vi "GetInfo.vi"(8 "error in (no error)":errorcluster caption="错误输入（无错误）", 11 "XYPlot 输入":refnum<class "TrendPlot.lvclass">) -> (0 "error out":errorcluster caption="错误输出", 2 "通道变更":bool, 3 "XYPlot 输出":refnum<class "TrendPlot.lvclass">)   [LabVIEW 2018, in "DataDisplay.lvlib" / "TrendPlot.lvclass"]
uses:
  TrendPlot.lvclass
  TrendPlot.lvclass/TrendPlot.ctl
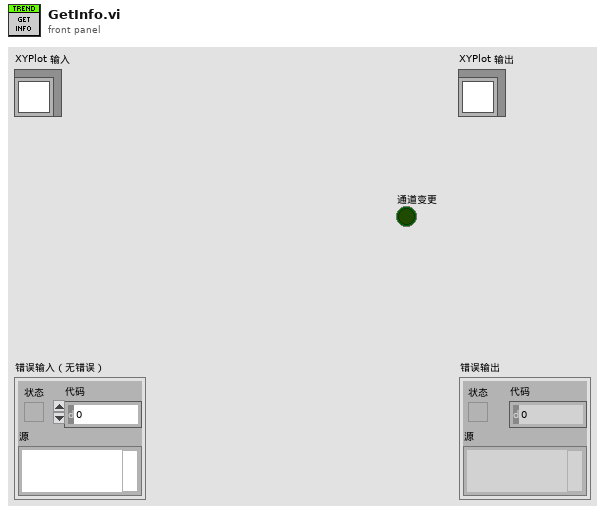
[diagram p1: front panel]
types:
  T1 = typedef "DataDisplay.lvlib/DD_CommandQ.ctl" = refnum<queue>
  T2 = typedef "DataDisplay.lvlib/DD_Command.ctl" = cluster{"消息":string, "参数":variant}
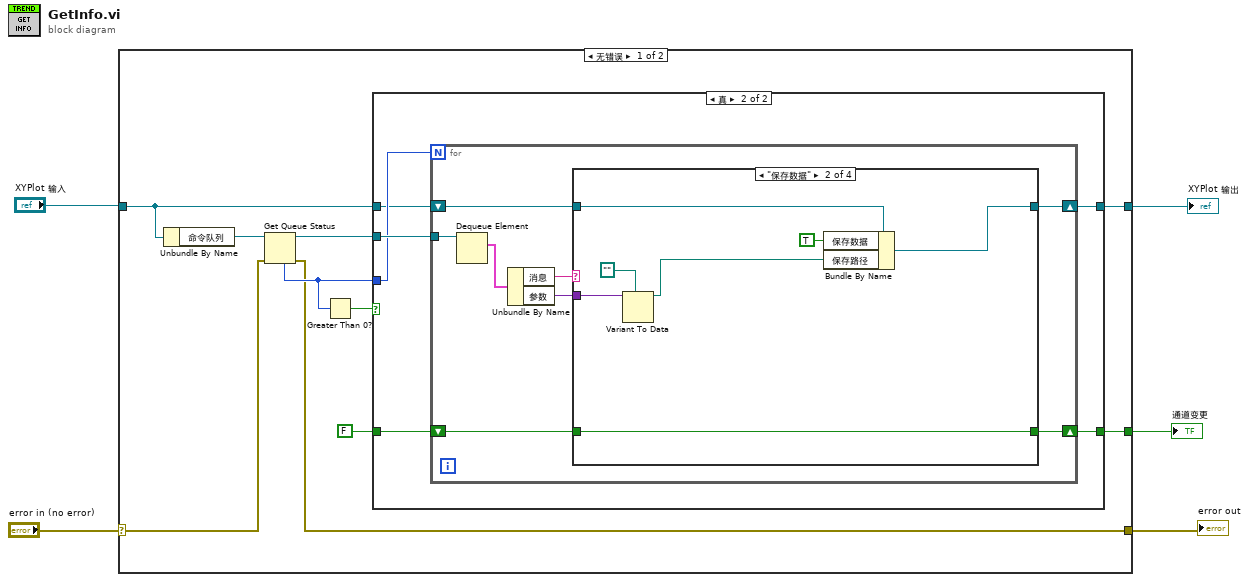
[diagram p0: block diagram]
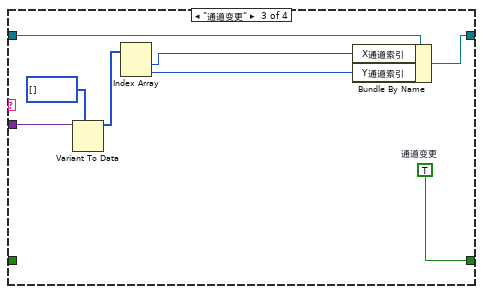
[diagram p4: hidden frame]
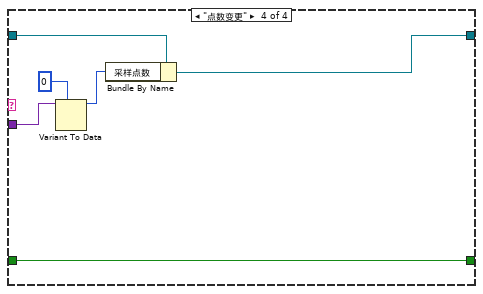
[diagram p5: hidden frame]
diagram:
  n1 = case shown="无错误" "error in (no error)" {
    selector: "error in (no error)" -> [w7 w56]
    tunnel: [w6 w56] -> w2
    tunnel: [w10 w55] -> w4
    tunnel: "XYPlot 输入" -> [w11 w55]
    tunnel: [w8 _] -> w1
    frame No Error {
      n2 = Unbundle By Name(w11) -> ("命令队列"=w15:T1)
      n3 = Get Queue Status(queue=w15, error in (no error)=w7) -> (queue out=w14:T1, error out=w6:errorcluster, # elements in queue=w13:i32)  [unwired: 1 in, 5 out]
      n4 = Greater Than 0?(x=w13) -> (x > 0?=w12:bool)
      n5 = case shown="真" w12 {
        tunnel: w14 -> [_ w23]
        tunnel: w13 -> [_ w22]
        tunnel: w11 -> [w17 w21]
        tunnel: [w17 w20] -> w10
        tunnel: [w16 w19] -> w8
        tunnel: FALSE -> [w16 w18]
        frame False {
        }
        frame True {
          n6 = for {
            N: w22 -> [_]
            tunnel: w23 -> [w31]
            shift-right: [w26] -> w20
            shift-left: w21 -> [w28]
            shift-right: [w24] -> w19
            shift-left: w18 -> [w25]
            n7 = Dequeue Element(queue=w31) -> (element=w30:T2)  [unwired: 2 in, 3 out]
            n8 = Unbundle By Name(w30) -> ("消息"=w29:string, "参数"=w27:variant)
            n9 = case shown="\"保存数据\"" w29 {
              tunnel: w28 -> [w33 w37 w41 w54]
              tunnel: w27 -> [_ w39 w48 w53]
              tunnel: [w33 w36 w45 w50] -> w26
              tunnel: w25 -> [w32 w40 _ w49]
              tunnel: [w32 w40 w42 w49] -> w24
              frame "假", Default {
              }
              frame "保存数据" {
                n10 = Variant To Data(type=path "", Variant=w39) -> (data=w35:path)  [unwired: 1 in, 1 out]
                n11 = Bundle By Name(cluster=w37, "保存数据"=TRUE, "保存路径"=w35) -> (w36:refnum<class "TrendPlot.lvclass">)
              }
              frame "通道变更" {
                w42 = TRUE  # 通道变更
                n12 = Variant To Data(type=i32[] [], Variant=w48) -> (data=w46:i32[])  [unwired: 1 in, 1 out]
                n13 = Index Array(array=w46) -> (element #1=w44:i32, element #2=w43:i32)  [unwired: 2 in]
                n14 = Bundle By Name(cluster=w41, "X通道索引"=w44, "Y通道索引"=w43) -> (w45:refnum<class "TrendPlot.lvclass">)
              }
              frame "点数变更" {
                n15 = Variant To Data(type=0, Variant=w53) -> (data=w52:i32)  [unwired: 1 in, 1 out]
                n16 = Bundle By Name(cluster=w54, "采样点数"=w52) -> (w50:refnum<class "TrendPlot.lvclass">)
              }
            }
          }
        }
      }
    }
    frame Error {
    }
  }
  "error out" <- w2
  "XYPlot 输出" <- w4
  "通道变更" <- w1
